vi "Pololu-Set Speed.vi"(4 "User Scale Max":u16, 5 "Servo Units Max":u16, 6 "User Scale Min":u16, 7 "Servo Units Min":u16, 8 "error in":errorcluster, 9 "Servo Chan":u16, 10 "Velocity (deg/sec)":u16, 11 "VISA resource name":refnum<visa-resource-name>) -> (0 "error out":errorcluster)   [LabVIEW 2018]
uses:
  <vilib>/Instr/_visa.llb/VISA Configure Serial Port (Instr).vi
panel:
  out "sent string":string
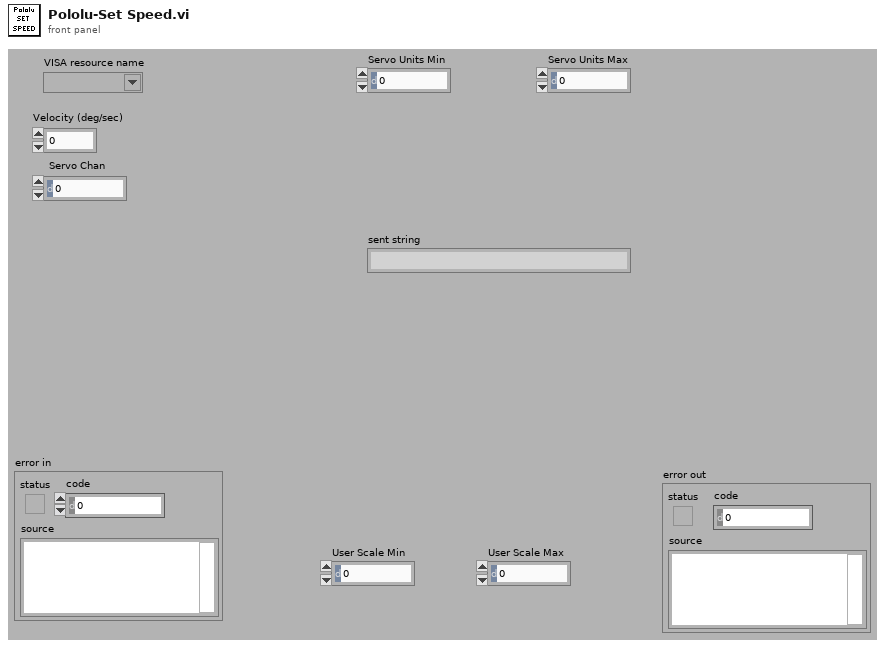
[diagram p1: front panel]
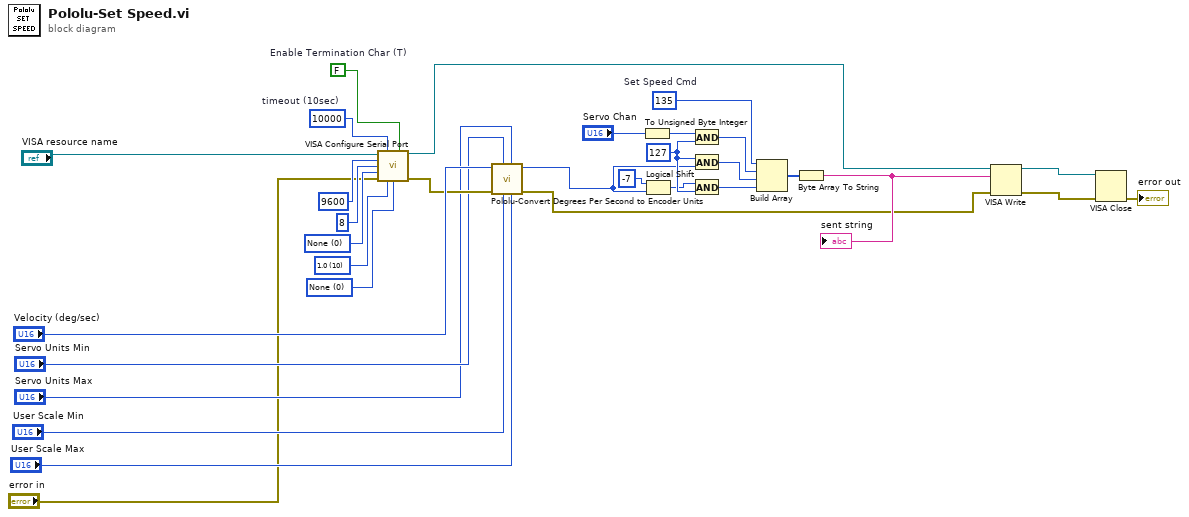
[diagram p0: block diagram]
diagram:
  w9 = u16 0 items=["None"=0, "XON/XOFF"=1, "RTS/CTS"=2, "DTR/DSR"=4] ("flow control")
  w10 = u16 10 items=["1.0"=10, "1.5"=15, "2.0"=20] ("stop bits")
  w11 = u16 0 items=["None", "Odd", "Even", "Mark", "Space"] ("parity")
  w14 = FALSE  # Enable Termination Char (T)
  w15 = u32 10000  # timeout (10sec)
  w24 = u8 135  # Set Speed Cmd
  w25 = u8 127
  n1 = call-poly "VISA Configure Serial Port"("VISA resource name"="VISA resource name", "timeout (10sec)"=w15, "Enable Termination\nChar (T)"=w14, "baud rate (9600)"=u32 9600 ("baud rate"), "data bits (8)"=u16 8 ("data bits"), "parity (0:none)"=w11, "error in (no error)"="error in", "stop bits (10: 1 bit)"=w10, "flow control (0:none)"=w9) -> ("VISA resource name out"=w29:refnum<visa-resource-name>, "error out"=w17:errorcluster)  [unwired: 5 out]
  n2 = call "Pololu-Convert Degrees Per Second to Encoder Units.vi"("Degree Max"="User Scale Max", "Encoder Units Max"="Servo Units Max", "Degree Min"="User Scale Min", "Encoder Units Min"="Servo Units Min", "Error In"=w17, "Speed (deg/sec)"="Velocity (deg/sec)") -> ("Error Out"=w16:errorcluster, "Speed Encoder Units"=w18:u16)  [unwired: 4 in]
  n3 = To Unsigned Byte Integer(number="Servo Chan") -> (unsigned 8bit integer=w4:u8)
  n4 = Logical Shift(y=i8 -7, x=w18) -> (x << y=w23:u16)
  n5 = And(x=w4, y=w25) -> (x .and. y?=w26:u8)
  n6 = And(x=w25, y=w18) -> (x .and. y?=w27:u16)
  n7 = And(x=w23, y=w25) -> (x .and. y?=w28:u16)
  n8 = Build Array(w24, w26, w27, w28) -> (w20:u16[])
  n9 = Byte Array To String(unsigned byte array=w20) -> (string=w21:string)
  "sent string" <- w21
  n10 = VISA Write(VISA resource name=w29, write buffer=w21, error in (no error)=w16) -> (VISA resource name out=w32:refnum<visa-resource-name>, error out=w31:errorcluster)  [unwired: 1 out]
  n11 = VISA Close(VISA resource name=w32, error in (no error)=w31) -> (error out=→"error out":errorcluster)
